vi "3d_mesh_test.vi"() -> ()   [LabVIEW 2016]
uses:
  <vilib>/picture/3D Picture Control/Object/Create Object (drawable with reference).vi
  <vilib>/picture/3D Picture Control/Object/Add Object (no reference).vi
  <vilib>/picture/3D Picture Control/Helpers/Set Light (reference).vi
  <vilib>/picture/3D Picture Control/NI_3D Picture Control.lvlib
panel:
  in  "Light State":enum16{"Inherit Value", "Off", "On"}(ring)=enum."On"
  in  "Vertex Array":T1(array[cluster])=[{"number: 0 to 1"=0.25, "number: 0 to 1"=0.25, "number: 0 to 1"=0.0}, {"number: 0 to 1"=0.75, "number: 0 to 1"=0.25, "number: 0 to 1"=0.25}, {"number: 0 to 1"=0.75, "number: 0 to 1"=0.75, "number: 0 to 1"=0.25}, {"number: 0 to 1"=0.25, "number: 0 to 1"=0.75, "number: 0 to 1"=0.0}, {"number: 0 to 1"=-0.25, "number: 0 to 1"=0.25, "number: 0 to 1"=0.0}, {"number: 0 to 1"=-0.25, "number: 0 to 1"=0.75, "number: 0 to 1"=0.0}, {"number: 0 to 1"=-0.75, "number: 0 to 1"=0.75, "number: 0 to 1"=0.25}, {"number: 0 to 1"=-0.75, "number: 0 to 1"=0.25, "number: 0 to 1"=0.25}, {"number: 0 to 1"=-0.25, "number: 0 to 1"=-0.25, "number: 0 to 1"=0.0}, {"number: 0 to 1"=-0.75, "number: 0 to 1"=-0.25, "number: 0 to 1"=0.25}, {"number: 0 to 1"=-0.75, "number: 0 to 1"=-0.75, "number: 0 to 1"=0.25}, {"number: 0 to 1"=-0.25, "number: 0 to 1"=-0.75, "number: 0 to 1"=0.0}, {"number: 0 to 1"=0.25, "number: 0 to 1"=-0.25, "number: 0 to 1"=0.0}, {"number: 0 to 1"=0.25, "number: 0 to 1"=-0.75, "number: 0 to 1"=0.0}, {"number: 0 to 1"=0.75, "number: 0 to 1"=-0.75, "number: 0 to 1"=0.25}, {"number: 0 to 1"=0.75, "number: 0 to 1"=-0.25, "number: 0 to 1"=0.25}] {"number: 0 to 1" scale=0.0..10.0; "number: 0 to 1" scale=0.0..10.0; "number: 0 to 1" scale=0.0..10.0}
  in  "Stop":bool
  out "3D Picture":refnum<vi>(3d-picture)
  in  "Light Direction":cluster{"X":sgl, "Y":sgl, "Z":sgl}={"X"=0.0, "Y"=0.0, "Z"=-1.0}
  in  "Light Colour":u32(colorbox)=16711680
  in  "Radius":sgl=0.01
  in  "Length":sgl=2.0
  in  "Character Size":sgl=0.5
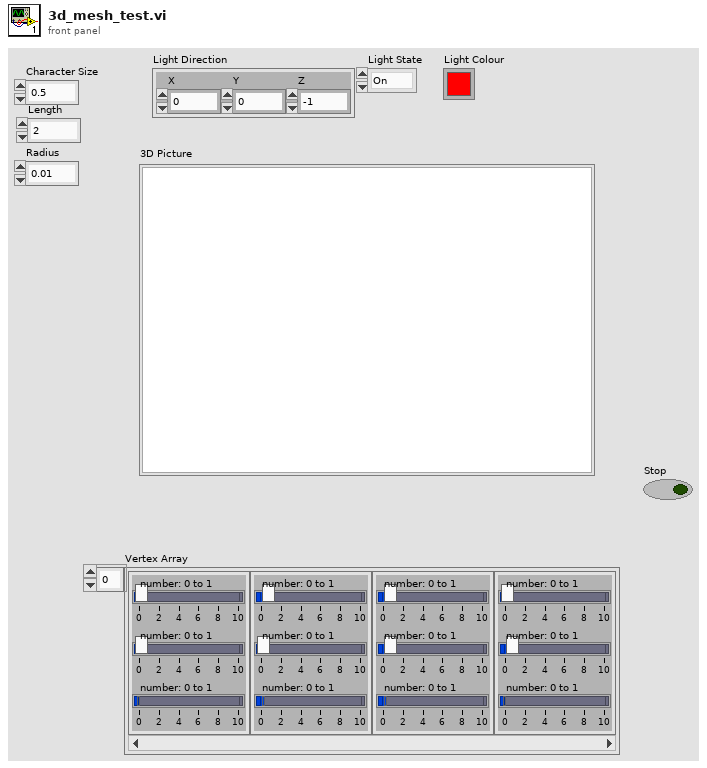
[diagram p1: front panel]
types:
  T1 = cluster{"number: 0 to 1":dbl, "number: 0 to 1":dbl, "number: 0 to 1":dbl}[]
  T2 = enum16{"Overall", "Per Primitive", "Per Vertex", "Binding Off"}
  T3 = enum16{"Points", "Lines", "Line Strip", "Line Loop", "Triangles", "Triangle Strip", "Triangle Fan", "Quads", "Quad Strip", "Polygon"}
  T4 = cluster{"number: 0 to 1":dbl, "number: 0 to 1":dbl, "number: 0 to 1":dbl, dbl}
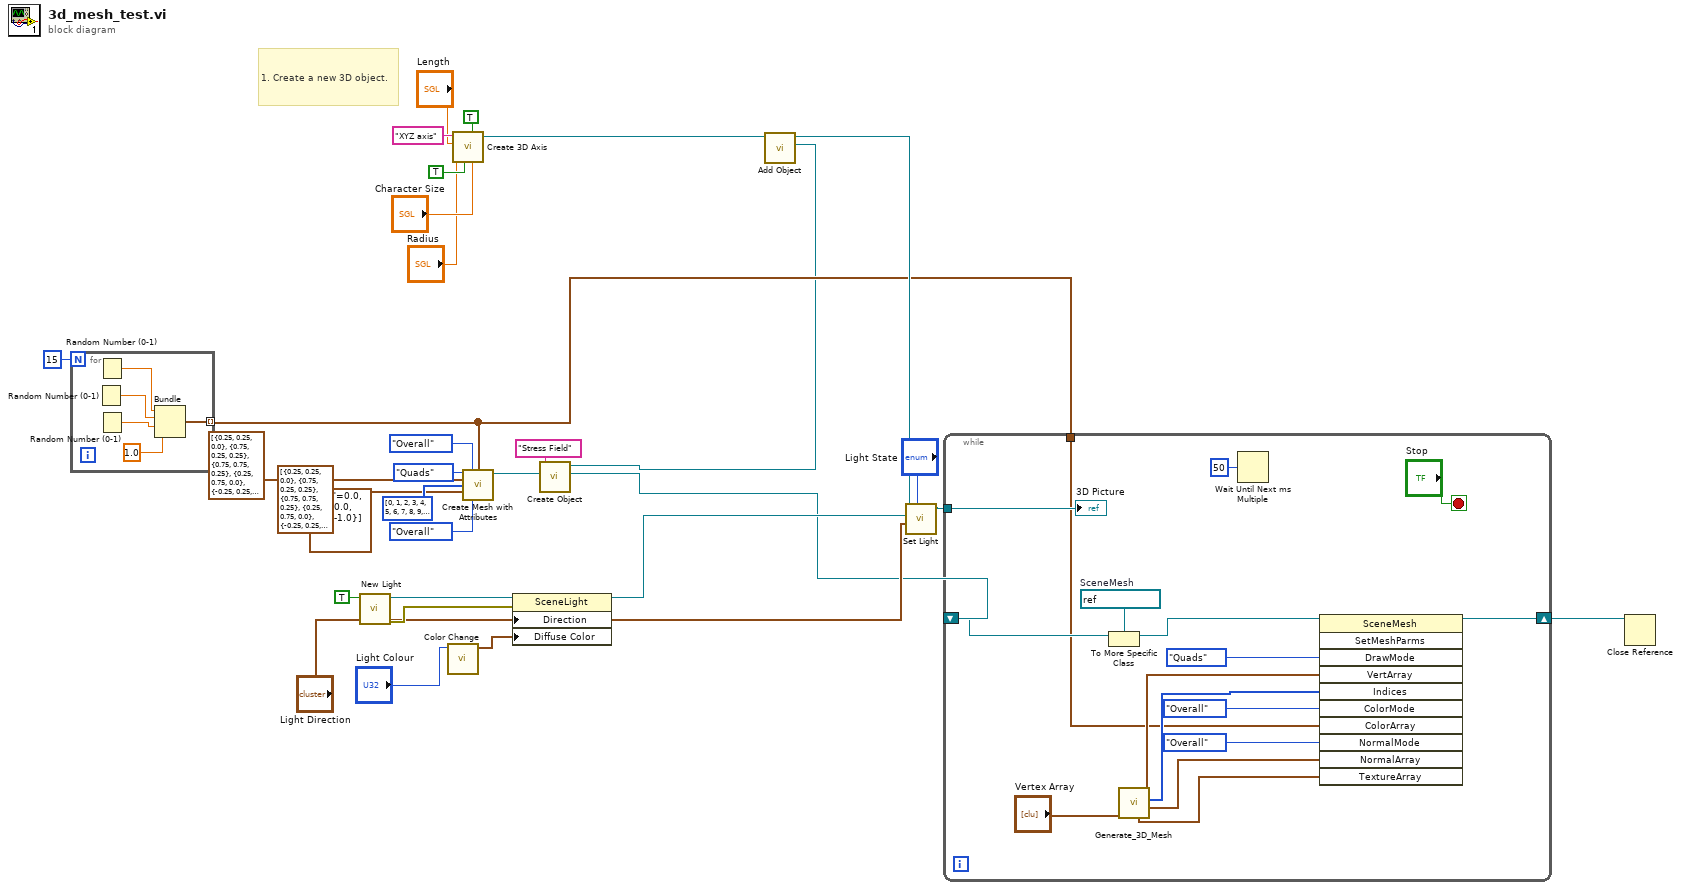
[diagram p0: block diagram]
diagram:
  (unwired) T1 [{"number: 0 to 1"=0.25, "number: 0 to 1"=0.25, "number: 0 to 1"=0.0}, {"number: 0 to 1"=0.75, "number: 0 to 1"=0.25, "number: 0 to 1"=0.25}, {"number: 0 to 1"=0.75, "number: 0 to 1"=0.75, "number: 0 to 1"=0.25}, {"number: 0 to 1"=0.25, "number: 0 to 1"=0.75, "number: 0 to 1"=0.0}, {"number: 0 to 1"=-0.25, "number: 0 to 1"=0.25, "number: 0 to 1"=0.0}, {"number: 0 to 1"=-0.25, "number: 0 to 1"=0.75, "number: 0 to 1"=0.0}, {"number: 0 to 1"=-0.75, "number: 0 to 1"=0.75, "number: 0 to 1"=0.25}, {"number: 0 to 1"=-0.75, "number: 0 to 1"=0.25, "number: 0 to 1"=0.25}, {"number: 0 to 1"=-0.25, "number: 0 to 1"=-0.25, "number: 0 to 1"=0.0}, {"number: 0 to 1"=-0.75, "number: 0 to 1"=-0.25, "number: 0 to 1"=0.25}, {"number: 0 to 1"=-0.75, "number: 0 to 1"=-0.75, "number: 0 to 1"=0.25}, {"number: 0 to 1"=-0.25, "number: 0 to 1"=-0.75, "number: 0 to 1"=0.0}, {"number: 0 to 1"=0.25, "number: 0 to 1"=-0.25, "number: 0 to 1"=0.0}, {"number: 0 to 1"=0.25, "number: 0 to 1"=-0.75, "number: 0 to 1"=0.0}, {"number: 0 to 1"=0.75, "number: 0 to 1"=-0.75, "number: 0 to 1"=0.25}, {"number: 0 to 1"=0.75, "number: 0 to 1"=-0.25, "number: 0 to 1"=0.25}] ("Vertex Array")
  # "1. Create a new 3D object."
  n1 = for {
    N: 15 -> [_]
    tunnel: [w35] -> w4 mode=indexing
    n2 = Random Number (0-1)() -> (number: 0 to 1=w32:dbl)
    n3 = Random Number (0-1)() -> (number: 0 to 1=w33:dbl)
    n4 = Random Number (0-1)() -> (number: 0 to 1=w31:dbl)
    n5 = Bundle("number: 0 to 1"=w33, "number: 0 to 1"=w32, "number: 0 to 1"=w31, 1.0) -> (w35:T4)  [unwired: 1 in]
  }
  n6 = call <vilib>:"New Light.vi"("At Infinity"=TRUE) -> ("error out"=w27:errorcluster, "New Light Refnum"=w30:refnum<vi>)  [unwired: 2 in, 7 out]
  n7 = call <vilib>:"Color Change.vi"("Color"="Light Colour") -> ("RGBA"=w26:cluster{"R":sgl, "G":sgl, "B":sgl, "A":sgl})  [unwired: 10 in]
  n8 = call <vilib>:"Create 3D Axis.vi"("Character Size"="Character Size", "Half plane?"=TRUE, "Axis label?"=TRUE, "Radius"="Radius", "Length"="Length", "Name"="XYZ axis") -> ("New Object Refnum"=w24:refnum<vi>)  [unwired: 4 in, 1 out]
  n9 = call <vilib>:"Create Mesh with Attributes.vi"("Draw Mode"=T3."Quads", "Color Binding Mode"=T2."Overall", "Color Array"=w4, "Vertex Array"=T1 [{"number: 0 to 1"=0.25, "number: 0 to 1"=0.25, "number: 0 to 1"=0.0}, {"number: 0 to 1"=0.75, "number: 0 to 1"=0.25, "number: 0 to 1"=0.25}, {"number: 0 to 1"=0.75, "number: 0 to 1"=0.75, "number: 0 to 1"=0.25}, {"number: 0 to 1"=0.25, "number: 0 to 1"=0.75, "number: 0 to 1"=0.0}, {"number: 0 to 1"=-0.25, "number: 0 to 1"=0.25, "number: 0 to 1"=0.0}, {"number: 0 to 1"=-0.25, "number: 0 to 1"=0.75, "number: 0 to 1"=0.0}, {"number: 0 to 1"=-0.75, "number: 0 to 1"=0.75, "number: 0 to 1"=0.25}, {"number: 0 to 1"=-0.75, "number: 0 to 1"=0.25, "number: 0 to 1"=0.25}, {"number: 0 to 1"=-0.25, "number: 0 to 1"=-0.25, "number: 0 to 1"=0.0}, {"number: 0 to 1"=-0.75, "number: 0 to 1"=-0.25, "number: 0 to 1"=0.25}, {"number: 0 to 1"=-0.75, "number: 0 to 1"=-0.75, "number: 0 to 1"=0.25}, {"number: 0 to 1"=-0.25, "number: 0 to 1"=-0.75, "number: 0 to 1"=0.0}, {"number: 0 to 1"=0.25, "number: 0 to 1"=-0.25, "number: 0 to 1"=0.0}, {"number: 0 to 1"=0.25, "number: 0 to 1"=-0.75, "number: 0 to 1"=0.0}, {"number: 0 to 1"=0.75, "number: 0 to 1"=-0.75, "number: 0 to 1"=0.25}, {"number: 0 to 1"=0.75, "number: 0 to 1"=-0.25, "number: 0 to 1"=0.25}], "Indices"=u32[] [0, 1, 2, 3, 4, 5, 6, 7, 8, 9, 10, 11, 12, 13, 14, 15], "Normal Array"=cluster{"X":sgl, "Y":sgl, "Z":sgl}[] [{"X"=0.0, "Y"=0.0, "Z"=-1.0}], "Normal Binding Mode"=T2."Overall") -> ("New Mesh Refnum"=w6:refnum<vi>)  [unwired: 7 in, 1 out]
  n10 = property class="SceneLight"(reference=w30, error in=w27, "Direction"="Light Direction", "Diffuse Color"=w26) -> (reference out=w7:refnum<vi>)  [unwired: 1 out]
  n11 = call-poly <vilib>:"Create Object.vi"("Geometry or text"=w6, "Name"="Stress Field") -> ("Drawable refnum"=w1:refnum<vi>, "Scene:New Object"=w2:refnum<vi>)  [unwired: 7 in, 1 out]
  n12 = call-poly <vilib>:"Add Object.vi"("New Object In"=w2, "Scene Object In"=w24) -> ("Scene Object Out"=w15:refnum<vi>)  [unwired: 8 in, 1 out]
  n13 = call-poly <vilib>:"Set Light.vi"("Light State"="Light State", "Position"="Light Direction", "Light Refnum In"=w7, "Scene Object In"=w15) -> ("Scene Object Out"=w14:refnum<vi>)  [unwired: 5 in, 2 out]
  n14 = while {
    tunnel: w14 -> [w51]
    tunnel: w4 -> [w39]
    shift-right: [w44] -> w5
    shift-left: w1 -> [w46]
    stop <- "Stop" stop-if-true
    w47 = refnum<vi> refnum  # SceneMesh
    n15 = To More Specific Class(target class=w47, reference=w46) -> (specific class reference=w45:refnum<vi>)  [unwired: 1 in, 1 out]
    n16 = call "Generate_3D_Mesh.vi"("XYZ Input"="Vertex Array") -> ("Normal Array"=w37:cluster{"X":sgl, "Y":sgl, "Z":sgl}[], "Indices"=w41:u32[], "Vertex Array"=w42:cluster{"X":sgl, "Y":sgl, "Z":sgl}[], "Texture Array"=w36:cluster{"X":sgl, "Y":sgl}[])  [unwired: 6 in, 1 out]
    n17 = Wait Until Next ms Multiple(millisecond multiple=u32 50) -> ()  [unwired: 1 out]
    n18 = invoke class="SceneMesh" method="SetMeshParms"(reference=w45, "DrawMode"=T3."Quads" ("Draw Mode"), "VertArray"=w42, "Indices"=w41, "ColorMode"=T2."Overall" ("Color Binding Mode"), "ColorArray"=w39, "NormalMode"=T2."Overall" ("Normal Binding Mode"), "NormalArray"=w37, "TextureArray"=w36) -> (reference out=w44:refnum<vi>)  [unwired: 2 in, 10 out]
    "3D Picture" <- w51
  }
  n19 = Close Reference(reference=w5) -> ()  [unwired: 1 in, 1 out]
